vi "Make an Array.vi"(8 "error in (no error)":errorcluster, 9 "Number of Dimensions":i32, 11 "Element Type":variant) -> (0 "error out":errorcluster, 3 "Array Type":variant)   [LabVIEW 2018, in "Scripting Tools.lvlib" / "XNode Support.lvlib"]
uses:
  XNode Support.lvlib
  <vilib>/Utility/VariantDataType/MemoryInfo.ctl
  <vilib>/Utility/VariantDataType/MemoryType.ctl
  <vilib>/Utility/VariantDataType/VariantType.lvlib
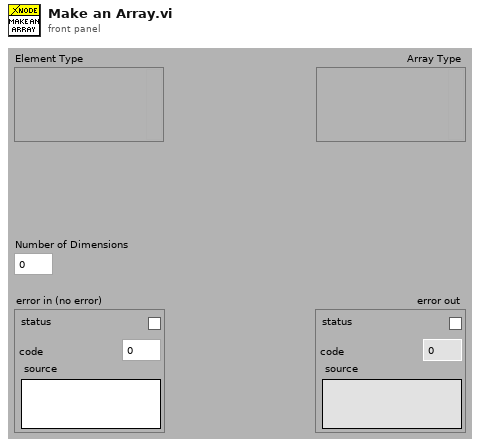
[diagram p1: front panel]
types:
  T1 = typedef "VariantType.lvlib/MemoryInfo.ctl" = cluster{"Type":T2, "Size":u32}
  T2 = typedef "VariantType.lvlib/MemoryType.ctl" = enum16{"Variable", "Fixed", "Bounded"}
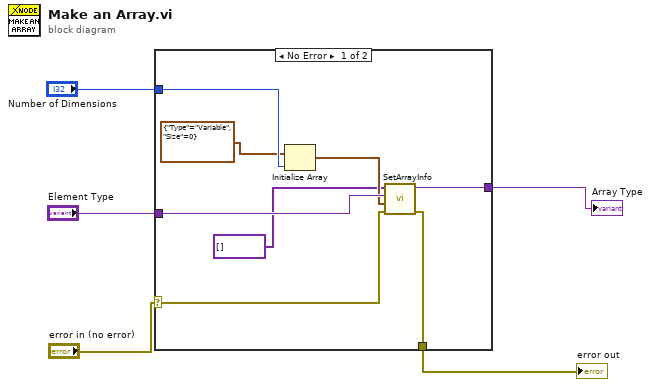
[diagram p0: block diagram]
diagram:
  n1 = case shown="No Error" "error in (no error)" {
    selector: "error in (no error)" -> [w8 w14]
    tunnel: "Element Type" -> [w13 _]
    tunnel: "Number of Dimensions" -> [w12 _]
    tunnel: [w9 _] -> w3
    tunnel: [w7 w14] -> w1
    frame No Error {
      n2 = Initialize Array(T1 {"Type"=enum."Variable", "Size"=0} ("MemoryType"), w12) -> (w10:T1[])
      n3 = call <vilib>:"SetArrayInfo.vi"("error in (no error)"=w8, "Array Lengths"=w10, "Array Element"=w13, "Variant"=variant[] []) -> ("error out"=w7:errorcluster, "Variant Out"=w9:variant)  [unwired: 6 out]
    }
    frame Error {
    }
  }
  "Array Type" <- w3
  "error out" <- w1
